vi "NISE.Execute Generic Command.vi"(0 "SLSC Interface in":refnum<class "SLSC Interface.lvclass">, 5 "resources":string, 7 "command":refnum<k21>, 11 "error in (no error)":errorcluster, 12 "timeout (10 sec)":dbl=10.0) -> (4 "SLSC Interface out":refnum<class "SLSC Interface.lvclass">, 15 "error out":errorcluster)   [LabVIEW 2016, in "SLSC Interface.lvclass"]
uses:
  SLSC Interface.lvclass
  SLSC Interface.lvclass/SLSC Interface.ctl
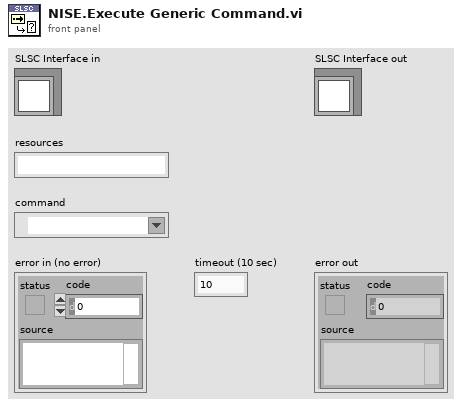
[diagram p1: front panel]
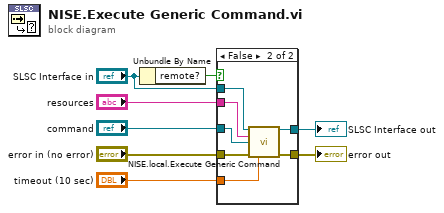
[diagram p0: block diagram]
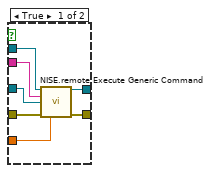
[diagram p2: hidden frame]
diagram:
  n1 = Unbundle By Name("SLSC Interface in") -> ("remote?"=w8:bool)
  n2 = case shown="False" w8 {
    tunnel: "SLSC Interface in" -> [w15 w22]
    tunnel: [w14 w21] -> w7
    tunnel: "resources" -> [w13 w20]
    tunnel: "command" -> [w12 w19]
    tunnel: "error in (no error)" -> [w11 w18]
    tunnel: "timeout (10 sec)" -> [w10 w17]
    tunnel: [w9 w16] -> w2
    frame True {
      n3 = call "NISE.remote.Execute Generic Command.vi"("SLSC Remote in"=w15, "resources"=w13, "command"=w12, "error in (no error)"=w11, "timeout (10 sec)"=w10) -> ("SLSC Remote out"=w14:refnum<class "SLSC Interface.lvclass">, "error out"=w9:errorcluster)  [unwired: 9 in]
    }
    frame False {
      n4 = call "NISE.local.Execute Generic Command.vi"("SLSC Local in"=w22, "resources"=w20, "command"=w19, "error in (no error)"=w18, "timeout (10 sec)"=w17) -> ("SLSC Local out"=w21:refnum<class "SLSC Interface.lvclass">, "error out"=w16:errorcluster)  [unwired: 9 in]
    }
  }
  "error out" <- w2
  "SLSC Interface out" <- w7
